vi "move.vi"(8 "error in (no error)":errorcluster, 11 "Mammal in":refnum<class "Mammal.lvclass">) -> (0 "error out":errorcluster, 2 "message":string, 3 "Mammal out":refnum<class "Mammal.lvclass">)   [LabVIEW 2017, in "Mammal.lvclass"]
uses:
  Mammal.lvclass
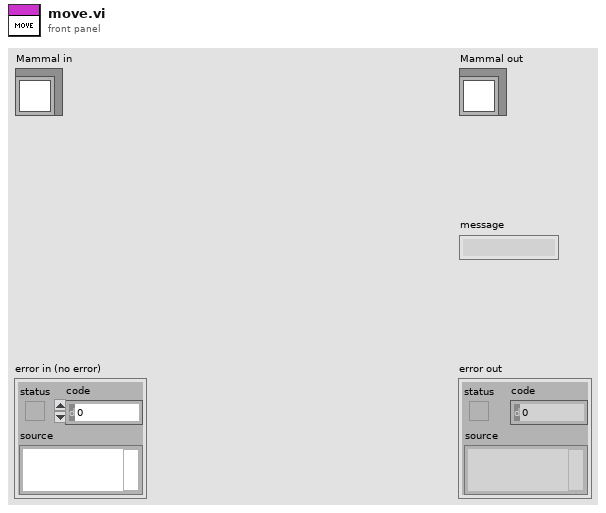
[diagram p1: front panel]
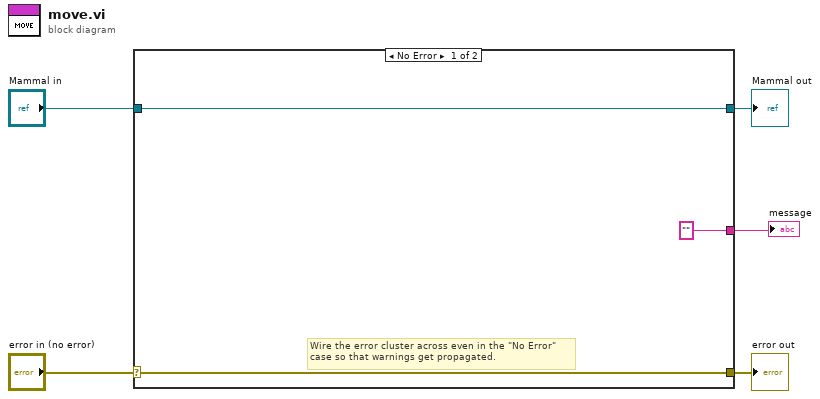
[diagram p0: block diagram]
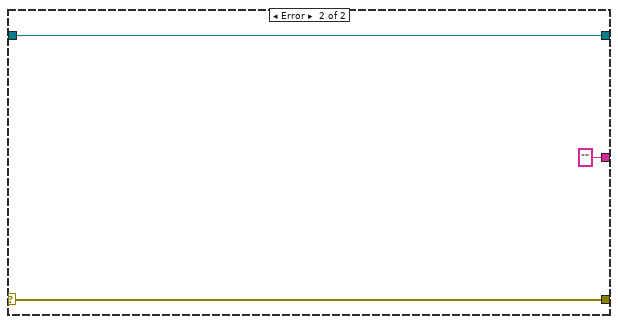
[diagram p2: hidden frame]
diagram:
  n1 = case shown="No Error" "error in (no error)" {
    selector: "error in (no error)" -> [w7 w11]
    tunnel: [w7 w11] -> w4
    tunnel: [w8 w10] -> w2
    tunnel: "Mammal in" -> [w8 w10]
    tunnel: ["" ""] -> w1
    frame No Error {
      # "Wire the error cluster across even in the \"No Error\"\ncase so that warnings get propagated."
    }
    frame Error {
    }
  }
  "error out" <- w4
  "Mammal out" <- w2
  "message" <- w1
